vi "AddHandler.vi"(8 "error in (no error)":errorcluster, 10 "Handler in":refnum<class "Handler.lvclass">, 11 "Logger in":refnum<class "Logger.lvclass">) -> (0 "error out":errorcluster, 2 "Handler out":refnum<class "Handler.lvclass">, 3 "Logger out":refnum<class "Logger.lvclass">)   [LabVIEW 2022 SP3, in "Logger.lvlib" / "Logger.lvclass"]
uses:
  Logger.lvclass
  C:/Users/jakub/repos/gh/PythonWrapper/Source/PythonWrapper/PythonWrapper.lvclass
  Handler/Handler.lvclass
  PythonWrapper/Source/PythonWrapper/PythonWrapper.lvclass/PythonWrapper.ctl
  Logger.lvclass/Logger.ctl
  Handler/Handler.lvclass/Handler.ctl
  Handler/Read Handler.vi
  PythonWrapper/Source/PythonWrapper/Read PythonSession.vi
  PythonWrapper/Source/PythonWrapper/Read ModulePath.vi
  Read Logger.vi
  Write Logger.vi
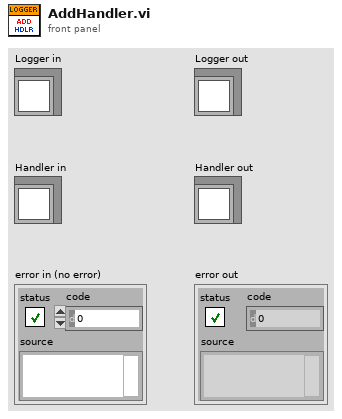
[diagram p1: front panel]
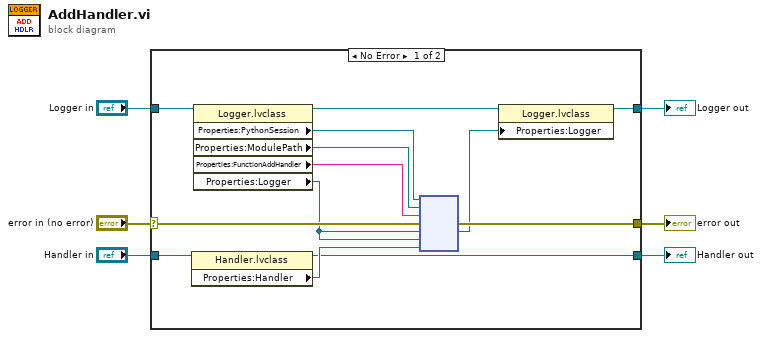
[diagram p0: block diagram]
diagram:
  n1 = case shown="No Error" "error in (no error)" {
    selector: "error in (no error)" -> [w17 w21]
    tunnel: [w16 w21] -> w3
    tunnel: [w10 w20] -> w5
    tunnel: "Logger in" -> [w19 w20]
    tunnel: "Handler in" -> [w11 _]
    tunnel: [w7 _] -> w1
    frame No Error {
      n2 = property class="Handler.lvclass"(reference=w11) -> (reference out=w7:refnum<class "Handler.lvclass">, "Properties:Handler"=w8:refnum<k38>)  [unwired: 1 in, 1 out]
      n3 = property class="Logger.lvclass"(reference=w19) -> (reference out=w18:refnum<class "Logger.lvclass">, "Properties:PythonSession"=w15:refnum<k35>, "Properties:ModulePath"=w13:path, "Properties:FunctionAddHandler"=w14:string, "Properties:Logger"=w12:refnum<k38>)  [unwired: 1 in, 1 out]
      n4 = node(w15, w13, w14, w17, w12, w12, w8) -> (w16:errorcluster, w9:refnum<k38>)  [unwired: 2 in, 3 out]
      n5 = property class="Logger.lvclass"(reference=w18, "Properties:Logger"=w9) -> (reference out=w10:refnum<class "Logger.lvclass">)  [unwired: 1 in, 1 out]
    }
    frame Error {
    }
  }
  "error out" <- w3
  "Logger out" <- w5
  "Handler out" <- w1
